vi "Joint Reference Follower (MS IOP).vi"(6 "Acc Ctrl Array":dbl[](array[numeric])=[0.0, 0.0, 0.0], 7 "Offset Home2RCM [deg/mm]":dbl[](array[numeric])=[0.0, 0.0, 0.0, 0.0], 8 "PID Ctrl Cluster":T1={"L1 PID Gains"={"Kp"=0.005, "Kd"=0.5, "Ki"=0.0005}, "L2 PID Gains"={"Kp"=0.01, "Kd"=1.0, "Ki"=0.005}, "L3 PID Gains"={"Kp"=0.05, "Kd"=1.0, "Ki"=0.0005}, "L4 PID Gains"={"Kp"=0.1, "Kd"=0.1, "Ki"=0.0005}}, 9 "Ref Array [deg/mm]":dbl[](array[numeric])=[0.0, 0.0, 0.0, 0.0], 10 "error in":errorcluster, 11 "FPGA VI Reference In":refnum<k20>) -> (1 "Output Posit Array [deg/mm]":dbl[](array[numeric]), 2 "error out":errorcluster, 3 "FPGA VI Reference Out":refnum<k20>)   [LabVIEW 2016]
uses:
  <vilib>/rvi/errors/niLvFpgaAdjustHostInterfaceError.vi
  <vilib>/Utility/error.llb/Error Cluster From Error Code.vi
  Subsystems/Global Variables.vi
  <vilib>/rvi/interface/nirviReadWriteControl/nirviReadWriteControl.xnode
  FPGA Bitfiles/PhantomControlPI_FPGATarget_QuadCtr2_E2412E44.lvbitx
  IRISS_FPGA_IO.vi
  Library/KevinLibraryAll/labview/KevLib01.lvlib
  NiFpgaLv.dll
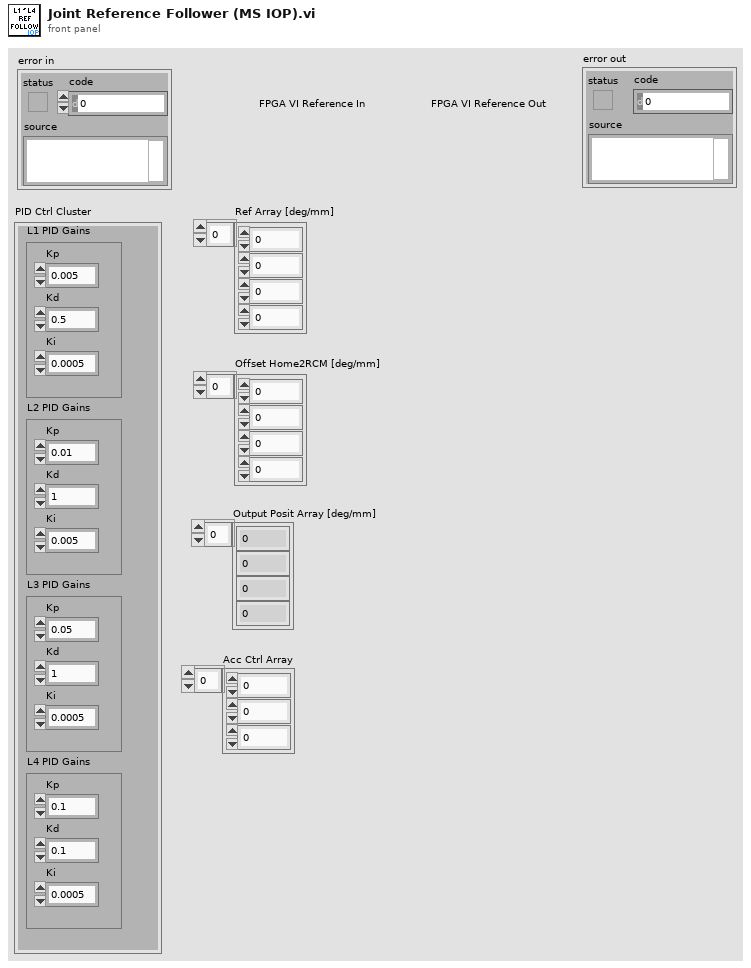
[diagram p1: front panel]
types:
  T1 = cluster{"L1 PID Gains":cluster{"Kp":dbl, "Kd":dbl, "Ki":dbl}, "L2 PID Gains":cluster{"Kp":dbl, "Kd":dbl, "Ki":dbl}, "L3 PID Gains":cluster{"Kp":dbl, "Kd":dbl, "Ki":dbl}, "L4 PID Gains":cluster{"Kp":dbl, "Kd":dbl, "Ki":dbl}}
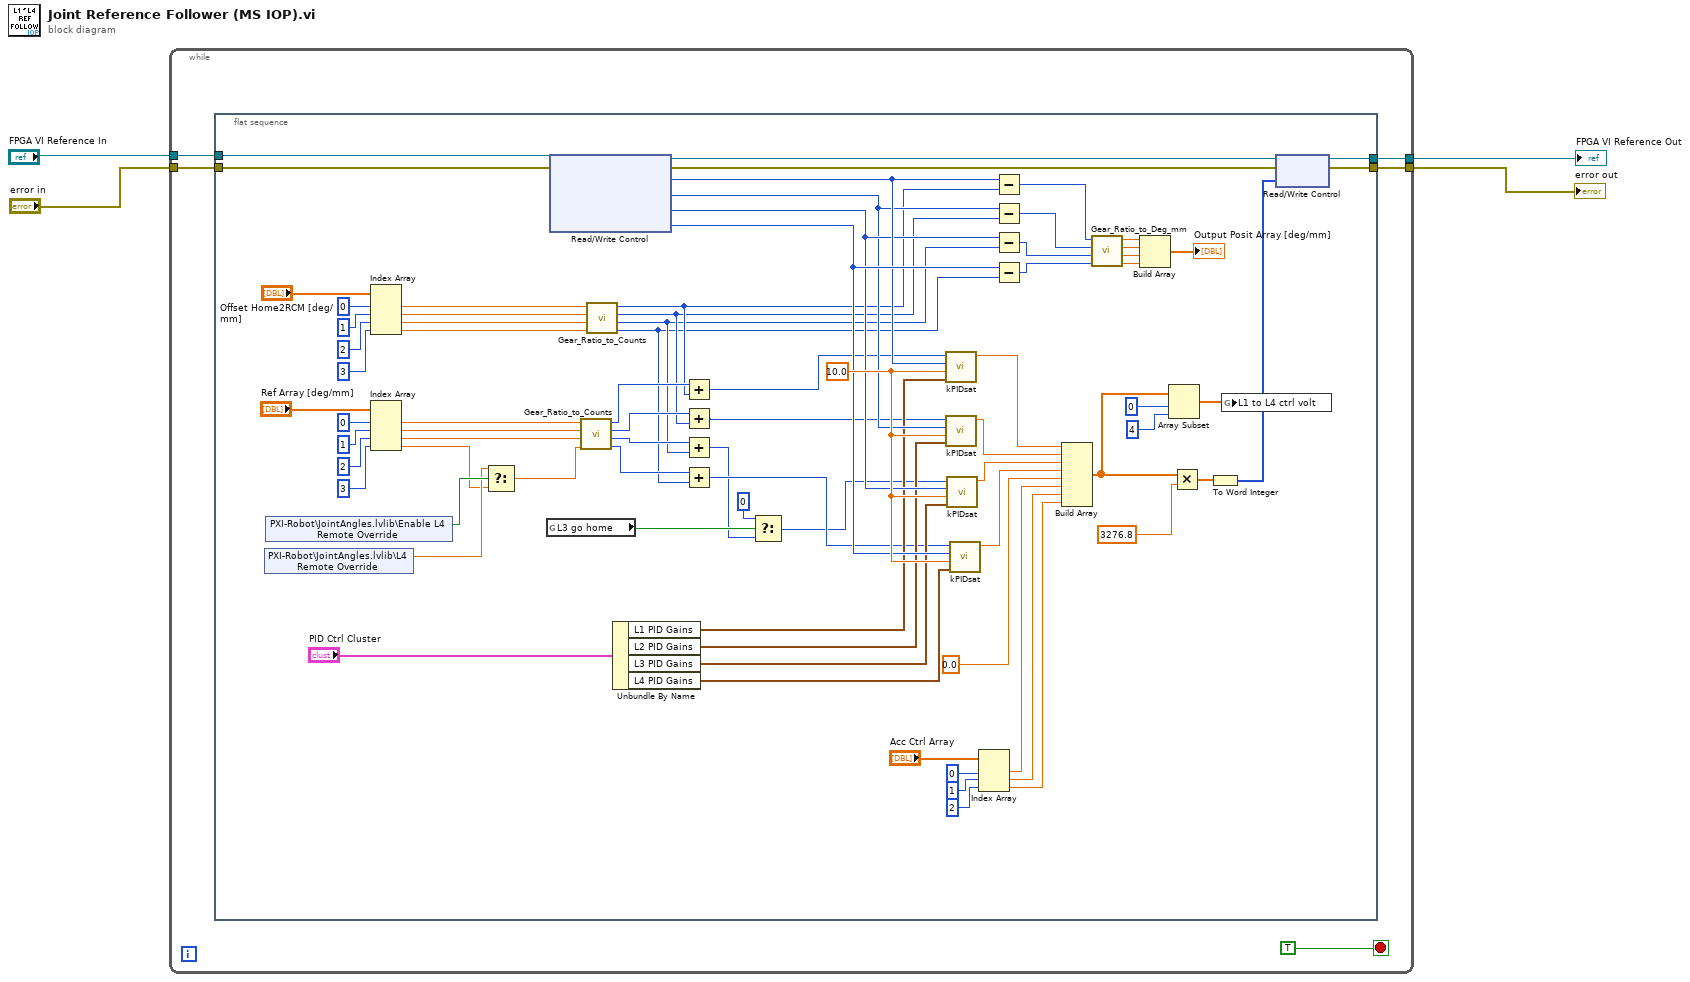
[diagram p0: block diagram]
diagram:
  n1 = while {
    tunnel: [w9] -> w1
    tunnel: [w8] -> w4
    tunnel: "FPGA VI Reference In" -> [w7]
    tunnel: "error in" -> [w6]
    stop <- TRUE ("Boolean") stop-if-true
    n2 = flat-sequence {
      tunnel: [w68] -> w9
      tunnel: [w67] -> w8
      tunnel: w7 -> [w45]
      tunnel: w6 -> [w44]
      frame #0 {
        w75 = 10.0 ("Sat Limit")
        n3 = shared-variable "PXI-Robot\\JointAngles.lvlib\\L4 Remote Override"() -> (w23:dbl)  [unwired: 1 in, 1 out]
        n4 = shared-variable "PXI-Robot\\JointAngles.lvlib\\Enable L4 Remote Override"() -> (w24:bool)  [unwired: 1 in, 1 out]
        n5 = Index Array(array="Offset Home2RCM [deg/mm]", index #1=0 ("index"), index #2=1 ("index"), index #3=2 ("index"), index #4=3 ("index")) -> (element #1=w43:dbl, element #2=w42:dbl, element #3=w41:dbl, element #4=w40:dbl)
        n6 = Index Array(array="Ref Array [deg/mm]", index #1=0 ("index"), index #2=1 ("index"), index #3=2 ("index"), index #4=3 ("index")) -> (element #1=w83:dbl, element #2=w82:dbl, element #3=w81:dbl, element #4=w22:dbl)
        n7 = Select(t=w23, s=w24, f=w22) -> (s? t:f=w21:dbl)
        n8 = global read "Global Variables.vi" "L3 go home"() -> (w28:bool)
        n9 = xnode "Read/Write Control"("FPGA VI Reference In"=w45, "error in"=w44) -> ("FPGA VI Reference Out"=w70:refnum<k20>, "error out"=w69:errorcluster, "32 bit Position 1"=w52:i32, "32 bit Position 3"=w50:i32, "32 bit Position C1-1"=w51:i32, "32 bit Position C1-4"=w62:i32)
        n10 = call "Gear_Ratio_to_Counts.vi"("theta 4"=w21, "theta 3"=w81, "theta 2"=w82, "theta 1"=w83) -> ("j4"=w33:i32, "j3"=w34:i32, "j2"=w35:i32, "j1"=w36:i32)
        n11 = call "Gear_Ratio_to_Counts.vi"("theta 4"=w40, "theta 3"=w41, "theta 2"=w42, "theta 1"=w43) -> ("j4"=w29:i32, "j3"=w30:i32, "j2"=w31:i32, "j1"=w32:i32)
        n12 = Unbundle By Name("PID Ctrl Cluster") -> ("L1 PID Gains"=w49:cluster{"Kp":dbl, "Kd":dbl, "Ki":dbl}, "L2 PID Gains"=w48:cluster{"Kp":dbl, "Kd":dbl, "Ki":dbl}, "L3 PID Gains"=w47:cluster{"Kp":dbl, "Kd":dbl, "Ki":dbl}, "L4 PID Gains"=w46:cluster{"Kp":dbl, "Kd":dbl, "Ki":dbl})
        n13 = Add(x=w36, y=w32) -> (x+y=w39:i32)
        n14 = Add(x=w35, y=w31) -> (x+y=w38:i32)
        n15 = Add(x=w34, y=w30) -> (x+y=w27:i32)
        n16 = Add(x=w33, y=w29) -> (x+y=w37:i32)
        n17 = Select(t=0 ("index"), s=w28, f=w27) -> (s? t:f=w25:i32)
        n18 = call "kPIDsat.vi"("PID Gains"=w49, "Sat Limit"=w75, "Position"=w52, "Reference"=w39) -> ("Control"=w61:dbl)  [unwired: 7 in]
        n19 = call "kPIDsat.vi"("PID Gains"=w48, "Sat Limit"=w75, "Position"=w50, "Reference"=w38) -> ("Control"=w63:dbl)  [unwired: 7 in]
        n20 = call "kPIDsat.vi"("PID Gains"=w47, "Sat Limit"=w75, "Position"=w51, "Reference"=w25) -> ("Control"=w64:dbl)  [unwired: 7 in]
        n21 = call "kPIDsat.vi"("PID Gains"=w46, "Sat Limit"=w75, "Position"=w62, "Reference"=w37) -> ("Control"=w74:dbl)  [unwired: 7 in]
        n22 = Index Array(array="Acc Ctrl Array", index #1=0 ("index"), index #2=1 ("index"), index #3=2 ("index")) -> (element #1=w16:dbl, element #2=w15:dbl, element #3=w14:dbl)
        n23 = Subtract(x=w52, y=w32) -> (x-y=w56:i32)
        n24 = Subtract(x=w50, y=w31) -> (x-y=w55:i32)
        n25 = Subtract(x=w51, y=w30) -> (x-y=w54:i32)
        n26 = Subtract(x=w62, y=w29) -> (x-y=w53:i32)
        n27 = Build Array(w61, w63, w64, w74, 0.0 ("element"), w16, w15, w14) -> (w13:dbl[])
        n28 = call "Gear_Ratio_to_Deg_mm.vi"("j4"=w53, "j3"=w54, "j2"=w55, "j1"=w56) -> ("theta 4"=w57:dbl, "theta 3"=w58:dbl, "theta 2"=w59:dbl, "theta 1"=w60:dbl)
        n29 = Build Array(w60, w59, w58, w57) -> (→"Output Posit Array [deg/mm]":dbl[])
        n30 = Array Subset(array=w13, index=0, length=4) -> (w18:dbl[])
        n31 = Multiply(x=w13, y=3276.8) -> (x*y=w72:dbl[])
        n32 = To Word Integer(number=w72) -> (16bit integer=w71:i16[])
        n33 = global write "Global Variables.vi" "L1 to L4 ctrl volt"(w18) -> ()
        n34 = xnode "Read/Write Control"("FPGA VI Reference In"=w70, "error in"=w69, "AO"=w71) -> ("FPGA VI Reference Out"=w68:refnum<k20>, "error out"=w67:errorcluster)
      }
    }
  }
  "error out" <- w4
  "FPGA VI Reference Out" <- w1
